vi "Round Floor to Places.vi"(9 "Places In":i32, 11 "Float In":sgl) -> (3 "Float Out":sgl format="%.1f")   [LabVIEW 2024, in "LVarex.lvlib"]
uses:
  LVarex.lvlib
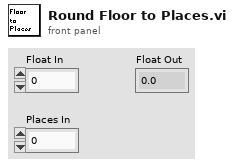
[diagram p1: front panel]
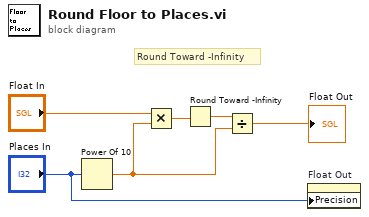
[diagram p0: block diagram]
diagram:
  # "Round Toward -Infinity"
  n1 = Power Of 10(x="Places In") -> (10^x=w3:dbl)
  n2 = Multiply(x="Float In", y=w3) -> (x*y=w5:dbl)
  n3 = Round Toward -Infinity(1:w5) -> (0:w4:dbl)
  n4 = Divide(x=w4, y=w3) -> (x/y=→"Float Out":dbl)
  n5 = property on="Float Out" class="DigNum (strict)"("Precision"="Places In") -> ()  [unwired: 2 in, 2 out]
